vi "read-file-data.vi"(8 "error in (no error)":errorcluster, 11 "dbc in":refnum<class "dbc.lvclass">) -> (0 "error out":errorcluster, 2 "dbc.data":T1, 3 "dbc out":refnum<class "dbc.lvclass">)   [LabVIEW 2015, in "dbc.lvclass"]
uses:
  dbc.lvclass
  controls/dbc-file-data.ctl
  dbc.lvclass/dbc.ctl
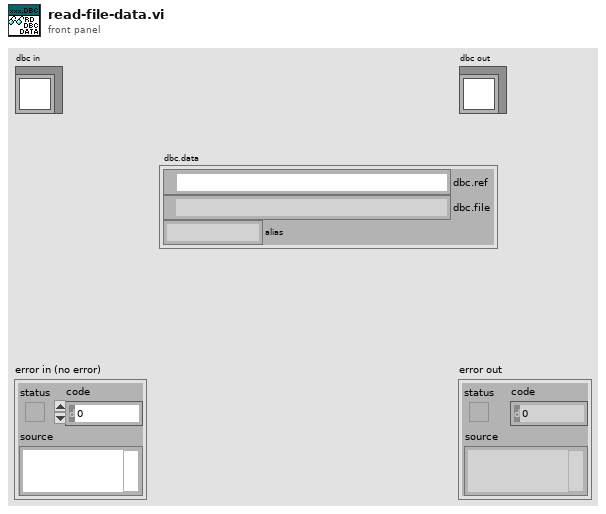
[diagram p1: front panel]
types:
  T1 = typedef "dbc-file-data.ctl" = cluster{"dbc.ref":refnum<k21>, "dbc.file":path, "alias":string}
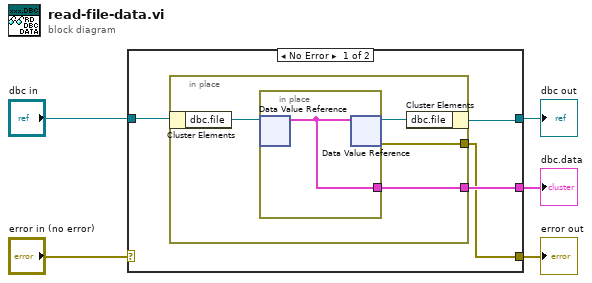
[diagram p0: block diagram]
diagram:
  n1 = case shown="No Error" "error in (no error)" {
    selector: "error in (no error)" -> [_ w15]
    tunnel: [w6 w15] -> w4
    tunnel: [w8 w16] -> w2
    tunnel: "dbc in" -> [w9 w16]
    tunnel: [w7 _] -> w1
    frame No Error {
      n2 = in-place {
        in-place-border: [w11] -> w6
        in-place-border: [w10] -> w7
        n3 = in-place-cluster #1(w9) -> ("dbc.file"=w13:refnum<data-value>)
        n4 = in-place {
          in-place-border: [w14] -> w10
          n5 = in-place-dvr #2(w13) -> (w14:T1)  [unwired: 1 out]
          n6 = in-place-dvr #2(w14) -> (w12:refnum<data-value>, w11:errorcluster)
        }
        n7 = in-place-cluster #1("dbc.file"=w12) -> (w8:refnum<class "dbc.lvclass">)
      }
    }
    frame Error {
    }
  }
  "error out" <- w4
  "dbc out" <- w2
  "dbc.data" <- w1
